vi "Stepper Control2.vi"() -> ()   [LabVIEW 2018]
uses:
  <vilib>/LabVIEW Interface for Arduino/Type Defs/Board Type.ctl
  <vilib>/LabVIEW Interface for Arduino/Type Defs/Connection Type.ctl
  <vilib>/LabVIEW Interface for Arduino/LabVIEW Interface for Arduino.lvlib
panel:
  out "ERROR":errorcluster
  in  "Baud Rate":u32=115200
  out "Step Angle":dbl
  in  "Step Size":i16
  out "Steps Remaining?":bool
  in  "Set Acceleration (0 to disable)":i16
  in  "Set Speed (Steps per Second)":i16=100
  in  "Steps for one rotation":i16
  in  "Control Method":u8(ring)=1 items=["2 Wire (Pulse & Direction)"=1, "2 Wire"=2, "4 Wire"=4, "EasyDriver"=6, "AF Motor Shield (Stepper 1 & 2 Only)"=5]
  in  "Stepper #":u8
  in  "error in":errorcluster
  in  "Board Type (Uno)":T1
  in  "VISA resource":refnum<visa-resource-name>
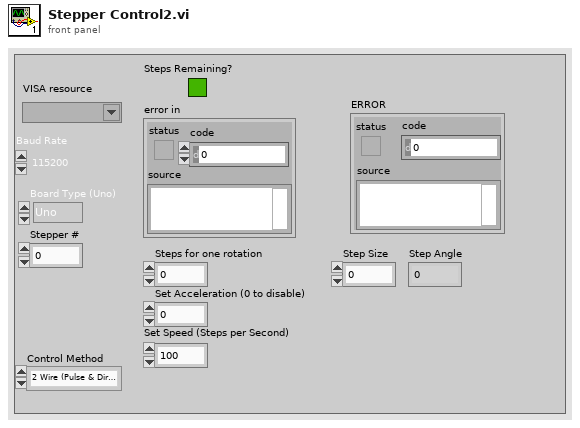
[diagram p1: front panel]
types:
  T1 = typedef "LabVIEW Interface for Arduino.lvlib/Board Type.ctl" = enum16{"Uno", "Dimuelanove w/Atmega 328", "Mega 2560"}
  T2 = typedef "LabVIEW Interface for Arduino.lvlib/Connection Type.ctl" = enum8{"USB / Serial", "XBEE", "BlueSmirf (Bluetooth)"}
  T3 = typedef "LabVIEW Interface for Arduino.lvlib/Arduino Resource.ctl" = cluster{"VISA resource":refnum<visa-resource-name>, "Board Type":T1, "Connection Type":enum8{"USB / Serial"}, "Bytes Per Packet (15)":u8}
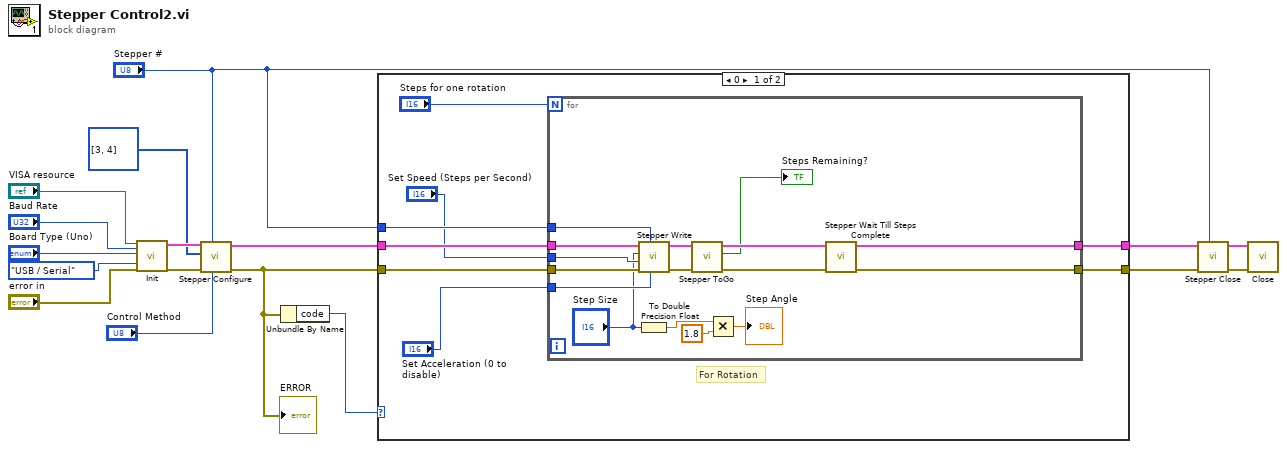
[diagram p0: block diagram]
diagram:
  n1 = call <vilib>:"Init.vi"("VISA resource"="VISA resource", "Baud Rate (115200)"="Baud Rate", "Board Type (Uno)"="Board Type (Uno)", "Connection Type (USB/Serial)"=Connection_Type."USB / Serial", "error in"="error in") -> ("Arduino Resource"=w14:T3, "error out"=w13:errorcluster)  [unwired: 13 in]
  n2 = call <vilib>:"Stepper Configure.vi"("Control Method"="Control Method", "Stepper #"="Stepper #", "error in"=w13, "Stepper Pins"=u8[] [3, 4], "Arduino Resource"=w14) -> ("error out"=w2:errorcluster, "Arduino Resource Out"=w4:T3)  [unwired: 5 in]
  "ERROR" <- w2
  n3 = Unbundle By Name(w2) -> ("code"=w1:i32)
  n4 = case shown="0" w1 {
    tunnel: [w25 w43] -> w7
    tunnel: [w24 w42] -> w6
    tunnel: "Stepper #" -> [w23 _]
    tunnel: w2 -> [w22 w43]
    tunnel: w4 -> [w21 w42]
    frame 0 {
      # "For Rotation"
      n5 = for {
        N: "Steps for one rotation" -> [_]
        tunnel: [w38] -> w25
        tunnel: [w37] -> w24
        tunnel: "Set Acceleration (0 to disable)" -> [w36]
        tunnel: w23 -> [w35]
        tunnel: w22 -> [w34]
        tunnel: "Set Speed (Steps per Second)" -> [w33]
        tunnel: w21 -> [w32]
        n6 = call <vilib>:"Stepper Write.vi"("Set Acceleration (0 to disable)"=w36, "Stepper #"=w35, "error in"=w34, "Set Speed (Steps per Second)"=w33, "# of Steps to Move"="Step Size", "Arduino Resource"=w32) -> ("error out"=w31:errorcluster, "Arduino Resource Out"=w30:T3)  [unwired: 4 in]
        n7 = To Double Precision Float(number="Step Size") -> (double precision float=w27:dbl)
        n8 = call <vilib>:"Stepper ToGo.vi"("error in"=w31, "Arduino Resource"=w30) -> ("error out"=w41:errorcluster, "Steps Remaining?"=→"Steps Remaining?":bool, "Arduino Resource Out"=w40:T3)  [unwired: 6 in, 1 out]
        n9 = Multiply(x=w27, y=1.8) -> (x*y=→"Step Angle":dbl)
        n10 = call <vilib>:"Stepper Wait Till Steps Complete.vi"("error in"=w41, "Arduino Resource In"=w40) -> ("error out"=w38:errorcluster, "Arduino Resource Out"=w37:T3)  [unwired: 8 in]
      }
    }
    frame 1, Default {
    }
  }
  n11 = call <vilib>:"Stepper Close.vi"("Stepper #"="Stepper #", "error in"=w7, "Arduino Resource"=w6) -> ("error out"=w8:errorcluster, "Arduino Resource Out"=w9:T3)  [unwired: 7 in]
  n12 = call <vilib>:"Close.vi"("Arduino Resource"=w9, "error in"=w8) -> ()  [unwired: 13 in, 1 out]
